vi "Set PostBuildAction VI.vi"(8 "error in (no error)":errorcluster, 10 "Project VI in":refnum<vi>, 11 "BuildSpec in":refnum<vi>) -> (0 "error out":errorcluster, 2 "Project VI out":refnum<vi>, 3 "BuildSpec out":refnum<vi>)   [LabVIEW 2019, in "Project Sync Tools.lvclass"]
uses:
  Project Sync Tools.lvclass
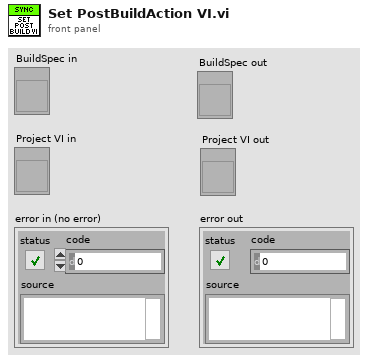
[diagram p1: front panel]
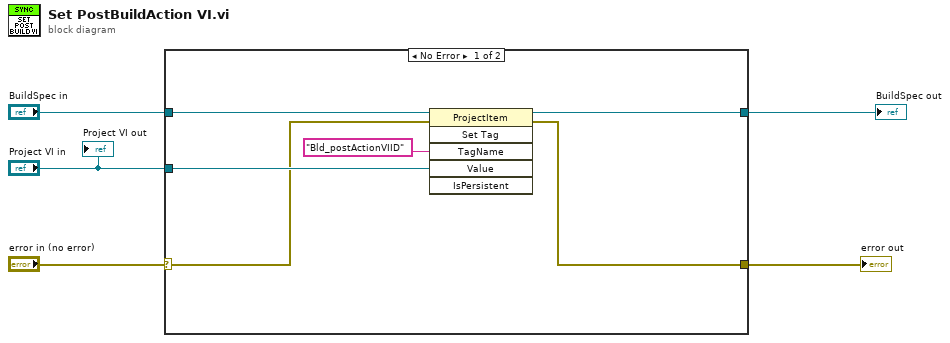
[diagram p0: block diagram]
diagram:
  n1 = case shown="No Error" "error in (no error)" {
    selector: "error in (no error)" -> [w6 w13]
    tunnel: [w11 w13] -> w5
    tunnel: [w10 w12] -> w4
    tunnel: "Project VI in" -> [w9 _]
    tunnel: "BuildSpec in" -> [w7 w12]
    frame No Error {
      n2 = invoke class="ProjectItem" method="Set Tag"(reference=w7, error in=w6, "TagName"="Bld_postActionVIID" ("Tag Name"), "Value"=w9) -> (reference out=w10:refnum<vi>, error out=w11:errorcluster)  [unwired: 2 in, 4 out]
    }
    frame Error {
    }
  }
  "error out" <- w5
  "BuildSpec out" <- w4
  "Project VI out" <- "Project VI in"
